vi "ListViewDemo.vi"() -> ()   [LabVIEW 2012]
uses:
  ListViewClass/ListViewClass.lvclass
  System.Windows.Forms
panel:
  in  "视图模式":i32(ring) items=["LargeIcon", "Details", "SmallIcon", "List", "Tile"]
  out "Selected Index":i32[](array[numeric])
  in  "Message":string
  in  "停止":bool
  in  "ListView":refnum<k24>(container)
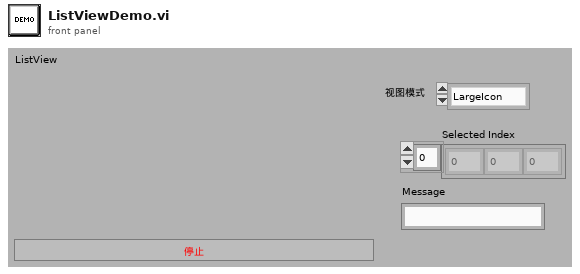
[diagram p1: front panel]
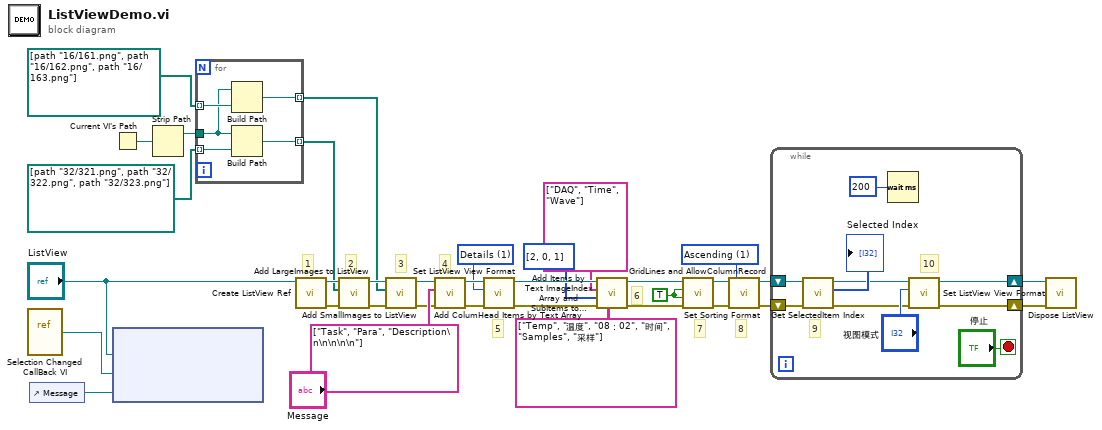
[diagram p0: block diagram]
diagram:
  w14 = TRUE ("GridLines")
  w30 = 1 items=["None", "Ascending", "Descending"] ("Sorting")
  w32 = 1 items=["LargeIcon", "Details", "SmallIcon", "List", "Tile"] ("View")
  # "8"
  # "7"
  # "6"
  # "5"
  # "4"
  # "3"
  # "2"
  # "1"
  n1 = vi-ref "Selection Changed CallBack VI.vi"() -> ("vi reference"=w11:refnum<vi>)
  n2 = control-ref of="Message"() -> (w12:refnum<vi>)
  n3 = Current VI's Path() -> (path=w8:path)
  n4 = node("ListView", w11, w12) -> ()  [unwired: 2 in, 2 out]
  n5 = Strip Path(path=w8) -> (stripped path=w7:path)  [unwired: 1 out]
  n6 = for {
    tunnel: w7 -> [w37]
    tunnel: path[] [path "16/161.png", path "16/162.png", path "16/163.png"] ("ImageFile Path") -> [w39] mode=indexing
    tunnel: path[] [path "32/321.png", path "32/322.png", path "32/323.png"] ("LargeImage") -> [w36] mode=indexing
    tunnel: [w38] -> w4 mode=indexing
    tunnel: [w35] -> w3 mode=indexing
    n7 = Build Path(base path=w37, name or relative path=w39) -> (appended path=w38:path)
    n8 = Build Path(base path=w37, name or relative path=w36) -> (appended path=w35:path)
  }
  n9 = call "Create ListView Ref.vi"("ListView"="ListView") -> ("error out"=w29:errorcluster, "ListViewClass 输出"=w28:refnum<class "ListViewClass.lvclass">)  [unwired: 9 in]
  n10 = call "Add LargeImages to ListView.vi"("error in (no error)"=w29, "LargeImage"=w3, "ListViewClass 输入"=w28) -> ("error out"=w24:errorcluster, "ListViewClass 输出"=w27:refnum<class "ListViewClass.lvclass">)  [unwired: 7 in]
  n11 = call "Add SmallImages to ListView.vi"("error in (no error)"=w24, "ImageFile Path"=w4, "ListViewClass 输入"=w27) -> ("error out"=w25:errorcluster, "ListViewClass 输出"=w26:refnum<class "ListViewClass.lvclass">)  [unwired: 7 in]
  n12 = call "Add ColumHead Items by Text Array.vi"("error in (no error)"=w25, "Text"=string[] ["Task", "Para", "Description\n\n\n\n\n"], "ListViewClass 输入"=w26) -> ("error out"=w31:errorcluster, "ListViewClass 输出"=w33:refnum<class "ListViewClass.lvclass">)  [unwired: 7 in]
  n13 = call "Set ListView View Format.vi"("error in (no error)"=w31, "View"=w32, "ListViewClass 输入"=w33) -> ("error out"=w22:errorcluster, "ListViewClass 输出"=w23:refnum<class "ListViewClass.lvclass">)  [unwired: 7 in]
  n14 = call "Add Items by Text ImageIndex Array and SubItems to ListView.vi"("SubItems"=string[][] [["Temp", "温度"], ["08：02", "时间"], ["Samples", "采样"]], "error in (no error)"=w22, "ImageIndex"=i32[] [2, 0, 1], "Text"=string[] ["DAQ", "Time", "Wave"], "ListViewClass 输入"=w23) -> ("error out"=w17:errorcluster, "ListViewClass 输出"=w18:refnum<class "ListViewClass.lvclass">)  [unwired: 5 in]
  n15 = call "GridLines and AllowColumnRecord.vi"("error in (no error)"=w17, "AllowColumnReorder"=w14, "GridLines"=w14, "ListViewClass 输入"=w18) -> ("error out"=w16:errorcluster, "ListViewClass 输出"=w15:refnum<class "ListViewClass.lvclass">)  [unwired: 6 in]
  n16 = call "Set Sorting Format.vi"("error in (no error)"=w16, "Sorting"=w30, "ListViewClass 输入"=w15) -> ("error out"=w20:errorcluster, "ListViewClass 输出"=w21:refnum<class "ListViewClass.lvclass">)  [unwired: 7 in]
  n17 = while {
    shift-right: [w40] -> w10
    shift-left: w21 -> [w48]
    shift-right: [w41] -> w9
    shift-left: w20 -> [w47]
    stop <- "停止" stop-if-true
    # "10"
    # "9"
    n18 = call "Get SelectedItem Index.vi"("error in (no error)"=w47, "ListViewClass 输入"=w48) -> ("error out"=w42:errorcluster, "Selected Index"=→"Selected Index":i32[], "ListViewClass 输出"=w44:refnum<class "ListViewClass.lvclass">)  [unwired: 7 in]
    n19 = Wait (ms)(milliseconds to wait=u32 200 ("等待时间（毫秒）")) -> ()  [unwired: 1 out]
    n20 = call "Set ListView View Format.vi"("error in (no error)"=w42, "View"="视图模式", "ListViewClass 输入"=w44) -> ("error out"=w41:errorcluster, "ListViewClass 输出"=w40:refnum<class "ListViewClass.lvclass">)  [unwired: 7 in]
  }
  n21 = call "Dispose ListView.vi"("error in (no error)"=w9, "ListViewClass 输入"=w10) -> ()  [unwired: 8 in, 2 out]
